vi "Keithley6514test.vi"   [LabVIEW 2015]
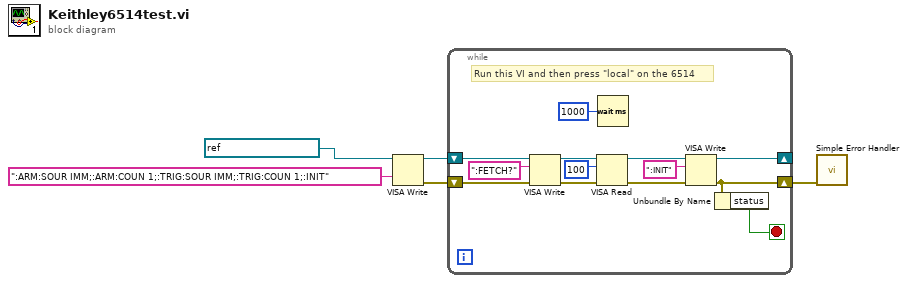
[diagram p0: block diagram]
diagram:
  n1 = VISA Write(VISA resource name=refnum<visa-resource-name> "GPIB0::14::INSTR", write buffer=":ARM:SOUR IMM;:ARM:COUN 1;:TRIG:SOUR IMM;:TRIG:COUN 1;:INIT") -> (VISA resource name out=w2:refnum<visa-resource-name>, error out=w3:errorcluster)  [unwired: 1 in, 1 out]
  n2 = while {
    shift-right: [w7] -> w1
    shift-left: w3 -> [w18]
    shift-right: [w8] -> _
    shift-left: w2 -> [w17]
    stop <- w6 stop-if-true
    # "Run this VI and then press \"local\" on the 6514"
    n3 = VISA Write(VISA resource name=w17, write buffer=":FETCH?", error in (no error)=w18) -> (VISA resource name out=w15:refnum<visa-resource-name>, error out=w14:errorcluster)  [unwired: 1 out]
    n4 = VISA Read(VISA resource name=w15, byte count=u32 100, error in (no error)=w14) -> (VISA resource name out=w11:refnum<visa-resource-name>, error out=w10:errorcluster)  [unwired: 2 out]
    n5 = Wait (ms)(milliseconds to wait=u32 1000) -> ()  [unwired: 1 out]
    n6 = VISA Write(VISA resource name=w11, write buffer=":INIT", error in (no error)=w10) -> (VISA resource name out=w8:refnum<visa-resource-name>, error out=w7:errorcluster)  [unwired: 1 out]
    n7 = Unbundle By Name(w7) -> ("status"=w6:bool)
  }
  n8 = call <vilib>:"Simple Error Handler.vi"("error in (no error)"=w1) -> ()  [unwired: 4 in, 5 out]
